vi "5.4-6.7.2-Where Server.vi"() -> ()   [LabVIEW 2010]
doc: "Creates a named service and listens on the first available port. Whenever a client connects to the service, it responds with a message containing joystick data. The VI can be stopped using the STOP button."
uses:
  5.0-Global.vi
  5.7-UDP/5.7 LabVIEW Errors.ctl
  6-OCU Neurons/6.0-Super Heart Beat.ctl
panel:
  out "Super Heart Beat":T1
  in  "error in 2":errorcluster={"status"=TRUE, "code"=0, "source"=""}
  out "error out  2":errorcluster
  in  "stop":bool
  out "Probably a hello string":string
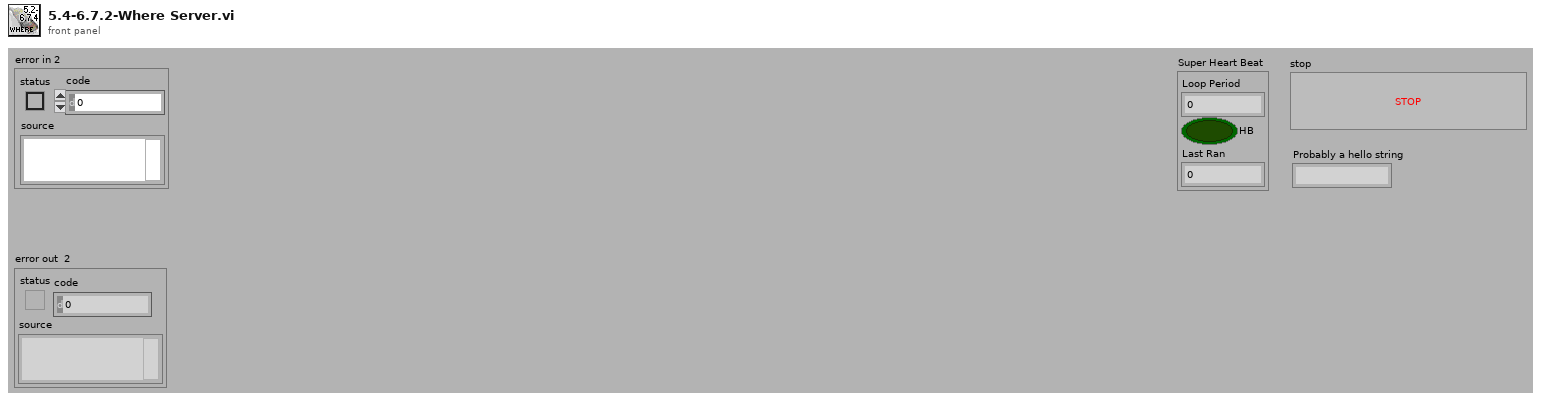
[diagram p1: front panel]
types:
  T1 = typedef "6.0-Super Heart Beat.ctl" = cluster{"Loop Period":u32, "HB":bool, "Last Ran":u32}
  T2 = typedef "6.2-Where Reporting.ctl" = cluster{"6.2 GPS Origin":cluster{"Lattitude (dd.mmmmmm)":ext, "Longitude (dd.mmmmmm)":ext}, "6.2 Where Data to Neo-Cortex":cluster{"X (Current)":dbl, "Y (Current) ":dbl, "Heading":dbl, "Steering Angle":dbl}, "6.2 MDF to Neo-Cortex":T3[]}
  T3 = typedef "MDF XY.ctl" = cluster{"Waypoint #":dbl, "X (waypoint)":ext, "Y  (waypoint)":ext, "Vel (desired)":dbl, "Dwell Time":dbl, "Behavior":enum16{"OpenFieldTransit", "WallFollow", "LaneFollow", "ManualMode"}, "Expand1":dbl, "Expand2":dbl, "Expand3":dbl}
  T4 = typedef "5.7 LabVIEW Errors.ctl" = i32
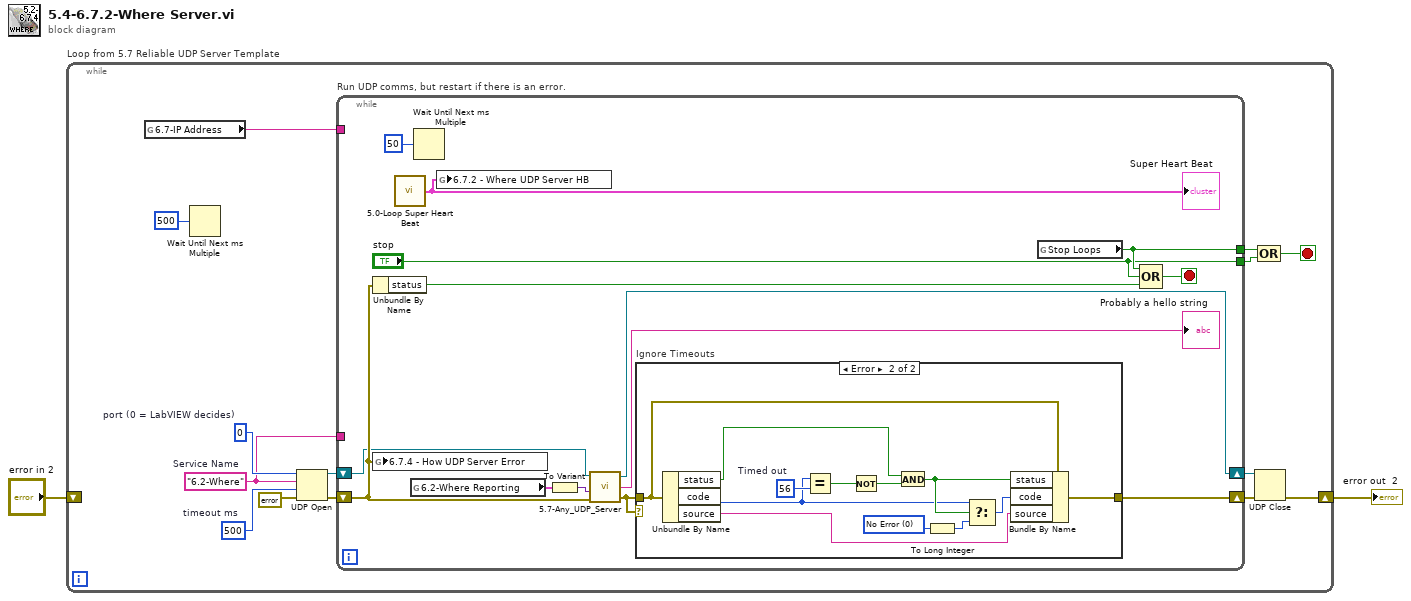
[diagram p0: block diagram]
diagram:
  n1 = while "Loop from 5.7 Reliable UDP Server Template" {
    shift-right: [w9] -> w1
    shift-left: "error in 2" -> [_]
    stop <- w14 stop-if-true
    w6 = 500  # timeout ms
    w8 = u16 0  # port (0 = LabVIEW decides)
    w7 = "6.2-Where"  # Service Name
    n2 = global read "5.0-Global.vi" "6.7-IP Address"() -> (w5:string)
    n3 = Wait Until Next ms Multiple(millisecond multiple=u32 500) -> ()  [unwired: 1 out]
    n4 = UDP Open(8:errorcluster {"status"=FALSE, "code"=0, "source"=""} ("error in (no error)"), 9:w6, 10:w7, 11:w8) -> (port=w13:refnum<k16>, 0:w11:errorcluster)  [unwired: 1 in, 1 out]
    n5 = while "Run UDP comms, but restart if there is an error." {
      tunnel: w7 -> [_]
      tunnel: w5 -> [_]
      tunnel: [w28] -> w16
      tunnel: ["stop"] -> w15
      shift-right: [w21] -> w12
      shift-left: w13 -> [w22]
      shift-right: [w25] -> w10
      shift-left: w11 -> [w24]
      stop <- w30 stop-if-true
      n6 = Unbundle By Name(w24) -> ("status"=w26:bool)
      n7 = global write "5.0-Global.vi" "6.7.4 - How UDP Server Error"(w24) -> ()
      n8 = call "5.0-Loop Super Heart Beat.vi"() -> ("Super Heart Beat"=w17:T1)
      "Super Heart Beat" <- w17
      n9 = global read "5.0-Global.vi" "6.2-Where Reporting"() -> (w18:T2)
      n10 = Wait Until Next ms Multiple(millisecond multiple=u32 50) -> ()  [unwired: 1 out]
      n11 = global write "5.0-Global.vi" "6.7.2 - Where UDP Server HB"(w17) -> ()
      n12 = To Variant(anything=w18) -> (Variant=w20:variant)
      n13 = call "5.7-Any_UDP_Server.vi"("error In"=w24, "Data in"=w20, "Connection ID"=w22) -> ("warning out"=w23:errorcluster, "data out"=→"Probably a hello string":string, "Connection ID out"=w21:refnum<k16>)  [unwired: 1 in]
      n14 = case "Ignore Timeouts" shown="Error" w23 {
        tunnel: w23 -> [w31 w43]
        tunnel: [w31 w42] -> w25
        frame No Error {
        }
        frame Error {
          w33 = T4 0 items=["No Error", "Argument Error", "Memory Full", "Out of Zone", "End of File", "File Already Open", "Generic File IO Error", "File Not Found", "File Permission Error", "Disk Full", "Duplicate Path", "Too Many Files Open", "Not Enabled", "Resource File Not Found", "Cannot Add Resource", "Resource Not Found", "Image Not Found", "Image Memory Error", "Pen Does Not Exist", "Config Bad Type", "Config Token Not Found", "Config Parse Error", "Config Memory Error", "Bad External Code Format", "Bad External Code Offset", "External Code Not Present", "Null Window", "Destroy Window Mixup", "Null Menu", "Print Aborted", "Bad Print Record", "Print Driver Error", "Windows Error During Print", "Memory Error During Print", "Print Dialog Error", "Generic Print Error", "Invalid Device Refnum", "Device Not Found", "Device Parameter Error", "Device Unit Error", "Can't Open Device", "Device Call Aborted", "Generic Error", "Cancelled By User", "Object ID Too Low", "Object ID Too High", "Object Not In Heap", "Unknown Heap", "Bad DefProc ID", "DefProc Not In Table", "Message Out Of Range", "Null Method", "Unknown Message", "Manager Call Not Supported", "Bad address", "Connection In progress", "Connection timed out", "Connection is already in progress", "Network attribute not supported", "Network error", "Address in use", "System out of memory", "Connection aborted", "Connection refused", "Connection is not connected", "Connection is already connected", "Connection closed", "Initialize error (interapplication manager)", "Bad occurrence", "Wait on unbound occurrence handler", "Occurrence queue overflow", "Bad path", "Semaphore not signaled", "Unrecognized type (interapplication manager)"] ("1st Error to Convert")
          w41 = 56  # Timed out
          n15 = Unbundle By Name(w43) -> ("status"=w38:bool, "code"=w36:i32, "source"=w34:string)
          n16 = Equal?(x=w36, y=w41) -> (x = y?=w40:bool)
          n17 = Not(x=w40) -> (.not. x?=w39:bool)
          n18 = And(x=w38, y=w39) -> (x .and. y?=w37:bool)
          n19 = To Long Integer(number=w33) -> (32bit integer=w32:T4)
          n20 = Select(t=w36, s=w37, f=w32) -> (s? t:f=w35:T4)
          n21 = Bundle By Name(cluster=w43, "status"=w37, "code"=w35, "source"=w34) -> (w42:errorcluster)
        }
      }
      n22 = global read "5.0-Global.vi" "Stop Loops"() -> (w28:bool)
      n23 = Compound Arithmetic op=OR(w28, "stop", w26) -> (w30:bool)
    }
    n24 = UDP Close(connection ID=w12, 8:w10) -> (error out=w9:errorcluster)  [unwired: 1 out]
    n25 = Compound Arithmetic op=OR(w16, w15) -> (w14:bool)
  }
  "error out  2" <- w1
